vi "sv_Get TDMS File Property Name String.vi"(7 "file properties":T1 items=["Enterprise", "Description", "Date and Time", "SV TDMS Format Version", "Alarm Detected?"]) -> (6 "property name":string, 8 "datatype":string)   [LabVIEW 2017]
uses:
  <vilib>/addons/_NISVFA/_Shared subVIs/Controls/NI File Properties.ctl
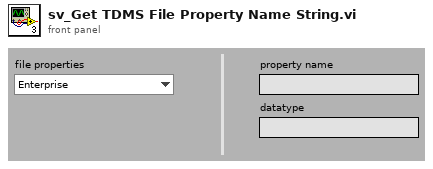
[diagram p1: front panel]
types:
  T1 = typedef "NI File Properties.ctl" = u16
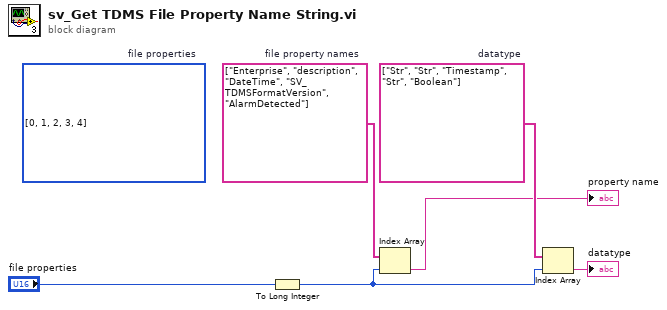
[diagram p0: block diagram]
diagram:
  (unwired) u16[] [0, 1, 2, 3, 4] items=["Enterprise", "Description", "Date and Time", "SV TDMS Format Version", "Alarm Detected?"]  # file properties
  w5 = string[] ["Str", "Str", "Timestamp", "Str", "Boolean"]  # datatype
  w6 = string[] ["Enterprise", "description", "DateTime", "SV_TDMSFormatVersion", "AlarmDetected"]  # file property names
  n1 = To Long Integer(number="file properties") -> (32bit integer=w1:i32)
  n2 = Index Array(array=w6, index=w1) -> (element=→"property name":string)
  n3 = Index Array(array=w5, index=w1) -> (element=→"datatype":string)
